vi "sub_log_scout.vi"(8 "error in":errorcluster, 11 "str":string) -> (0 "error out":errorcluster)   [LabVIEW 2019]
uses:
  logfile-name.vi
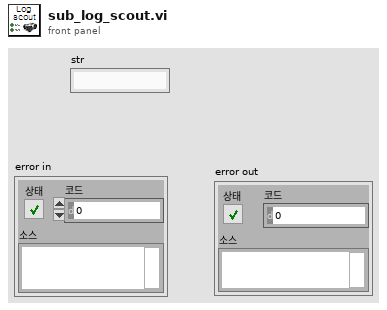
[diagram p1: front panel]
types:
  T1 = enum16{"open", "replace", "create", "open or create", "replace or create", "replace or create with confirmation"}
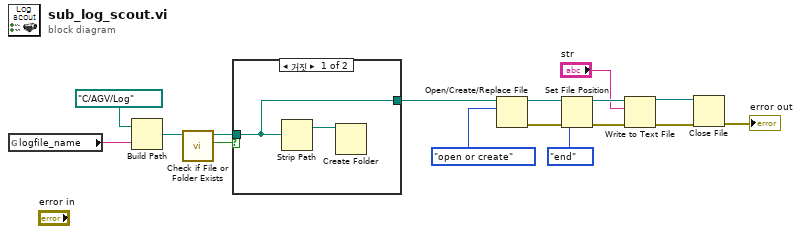
[diagram p0: block diagram]
diagram:
  n1 = global read "logfile-name.vi" "logfile_name"() -> (w1:string)
  n2 = Build Path(base path=path "C:/AGV/Log" ("베이스 경로"), name or relative path=w1) -> (appended path=w4:path)
  n3 = call <vilib>:"Check if File or Folder Exists.vi"("path"=w4) -> ("file or folder exists?"=w5:bool, "dup path"=w15:path)  [unwired: 8 in, 1 out]
  n4 = case shown="거짓" w5 {
    tunnel: w15 -> [w17 w19]
    tunnel: [w17 w19] -> w3
    frame False {
      n5 = Strip Path(path=w17) -> (stripped path=w18:path)  [unwired: 1 out]
      n6 = Create Folder(path (use dialog)=w18) -> ()  [unwired: 2 in, 3 out]
    }
    frame True {
    }
  }
  n7 = Open/Create/Replace File(file path (use dialog)=w3, operation (0:open)=T1."open or create" ("동작(0:open)")) -> (refnum out=w13:refnum<file>, error out=w12:errorcluster)  [unwired: 4 in, 1 out]
  n8 = Set File Position(refnum=w13, from (0:start)=enum16{"start", "end", "current"}."end" ("위치(0:start)"), error in=w12) -> (refnum out=w9:refnum<file>, error out=w10:errorcluster)  [unwired: 1 in]
  n9 = Write to Text File(file (use dialog)=w9, text="str", error in=w10) -> (refnum out=w7:refnum<file>, error out=w8:errorcluster)  [unwired: 1 in, 1 out]
  n10 = Close File(refnum=w7, error in=w8) -> (error out=→"error out":errorcluster)  [unwired: 1 out]
